vi "ReadSignals.Compile.vi"(8 "error in (no error)":errorcluster, 9 "Frame Settings Array":T4[](array[typedef]) {"Signals"."Byte Order" items=["Little Endian", "Big Endian"]; "Signals"."Data Type" items=["Signed", "Unsigned", "IEEE Float"]}, 10 "Refs":T3[](array[typedef]) {"Signal Refs" format="%.0x"}, 11 "Lookups in":variant) -> (0 "error out":errorcluster, 2 "Refs":T2 {"VS Refs" format="%.0x"}, 3 "Lookups":variant)   [LabVIEW 2019, in "Diagnostics Addon System Explorer.lvlib"]
uses:
  Diagnostics Addon System Explorer.lvlib
  Shared/Types/Frame.Compile.ctl
  Shared/Types/Type.ctl
  Shared/Types/Signal.ctl
  Types/Frame.Ref.ctl
  <vilib>/NI VeriStand/Custom Device API/Custom Device Item Ref.ctl
  Shared/Types/Frame.Lookup.Info.ctl
  Shared/SubVIs/Constants.vi
  Shared/Diagnostics Addon Shared.lvlib
  <vilib>/NI VeriStand/Custom Device API/Custom Device API.lvlib
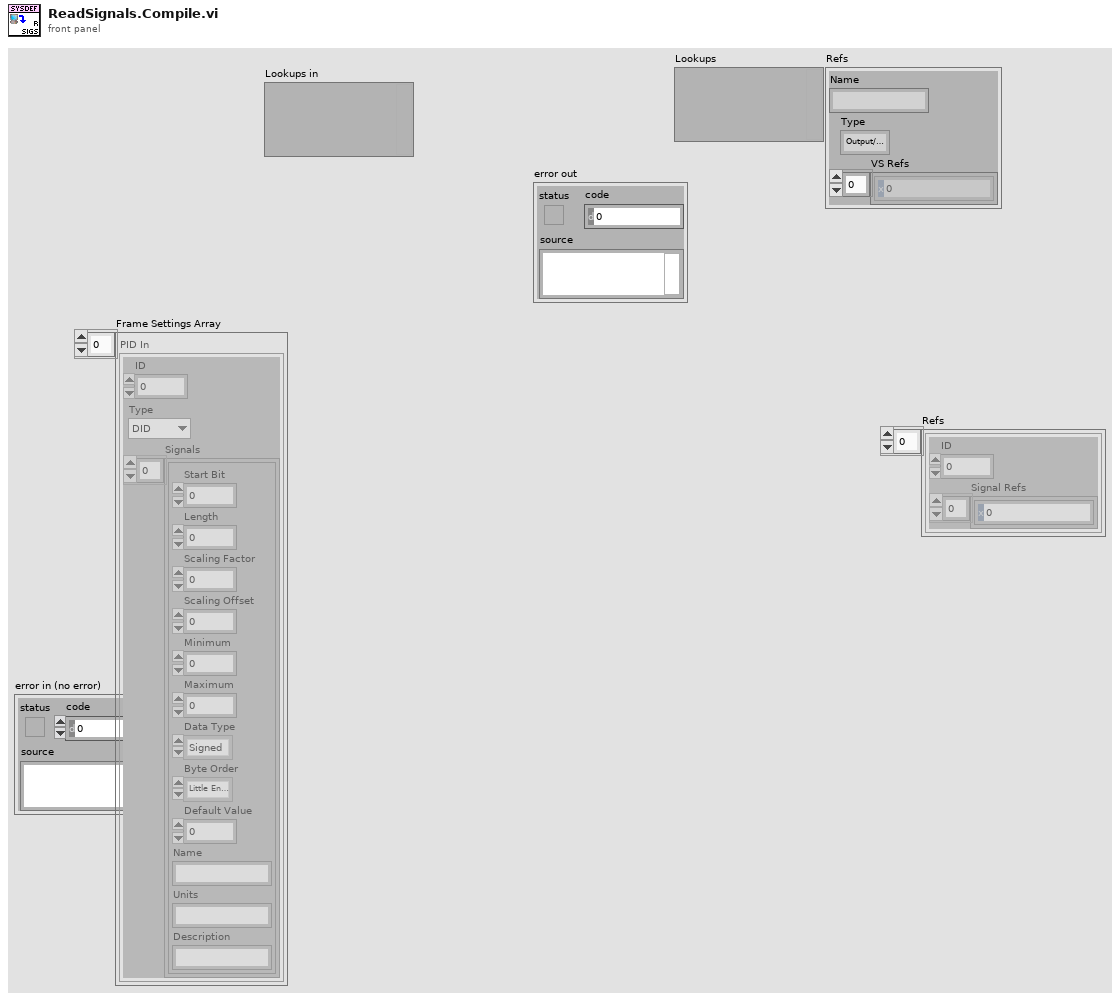
[diagram p1: front panel]
types:
  T1 = typedef "Custom Device API.lvlib/Custom Device Item Ref.ctl" = u64
  T2 = cluster{"Name":string, "Type":enum16{"Output/Write", "Input/Read", "Input/ReadWrite"}, "VS Refs":T1[]}
  T3 = typedef "Diagnostics Addon System Explorer.lvlib/Frame.Ref.ctl" = cluster{"ID":u32, "Signal Refs":T1[]}
  T4 = typedef "Diagnostics Addon Shared.lvlib/Frame.Compile.ctl" = cluster{"ID":u32, "Type":T5, "Signals":T6[]}
  T5 = typedef "Diagnostics Addon Shared.lvlib/Type.ctl" = enum16{"DID", "CDID", "PID", "CPID", "Read Memory", "Write Memory", "DTC Control", "IO Cmd", "IO Resp", "Routine Start Cmd", "Routine Start Resp", "Routine Request Cmd", "Routine Request Resp", "Routine Stop Cmd", "Routine Stop Resp", "UserDefined Cmd", "UserDefined Rsp"}
  T6 = typedef "Diagnostics Addon Shared.lvlib/Signal.ctl" = cluster{"Start Bit":u32, "Length":u32, "Scaling Factor":dbl, "Scaling Offset":dbl, "Minimum":dbl, "Maximum":dbl, "Data Type":u32, "Byte Order":u32, "Default Value":dbl, "Name":string, "Units":string, "Description":string}
  T7 = enum16{"Output/Write", "Input/Read", "Input/ReadWrite"}
  T8 = typedef "Diagnostics Addon Shared.lvlib/Frame.Lookup.Info.ctl" = cluster{"Offset":i32, "Length":i32, "ByteLength":u16}
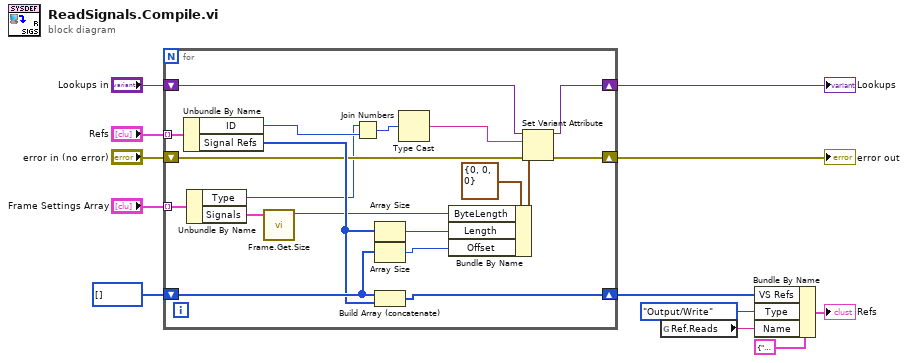
[diagram p0: block diagram]
diagram:
  n1 = for {
    tunnel: "Refs" -> [w21] mode=indexing
    shift-right: [w30] -> w3
    shift-left: T1[] [] ("Signal Refs") -> [w31]
    shift-right: [w22] -> w10
    shift-left: "Lookups in" -> [w26]
    shift-right: [w24] -> w1
    shift-left: "error in (no error)" -> [w19]
    tunnel: "Frame Settings Array" -> [w18] mode=indexing
    n2 = Unbundle By Name(w21) -> ("ID"=w15:u32, "Signal Refs"=w20:T1[])
    n3 = Unbundle By Name(w18) -> ("Type"=w13:T5, "Signals"=w17:T6[])
    n4 = call "Frame.Get.Size.vi"("Parameters"=w17) -> ("Bytes"=w16:u32)  [unwired: 10 in]
    n5 = Join Numbers(hi=w13, lo=w15) -> ((hi.lo)=w14:u64)
    n6 = Array Size(array=w20) -> (size(s)=w29:i32)
    n7 = Array Size(array=w31) -> (size(s)=w25:i32)
    n8 = Build Array (concatenate)(w31, w20) -> (w30:T1[])
    n9 = Type Cast(x=w14) -> (*(type *) &x=w23:string)  [unwired: 1 in]
    n10 = Bundle By Name(cluster=T8 {"Offset"=0, "Length"=0, "ByteLength"=0}, "ByteLength"=w16, "Length"=w29, "Offset"=w25) -> (w27:T8)
    n11 = Set Variant Attribute(Variant=w26, name=w23, value=w27, error in=w19) -> (Variant out=w22:variant, error out=w24:errorcluster)  [unwired: 1 out]
  }
  "error out" <- w1
  "Lookups" <- w10
  n12 = global read "Constants.vi" "Ref.Reads"() -> (w5:string)
  n13 = Bundle By Name(cluster=T2 {"Name"="", "Type"=enum."Output/Write", "VS Refs"=[]} ("Group"), "VS Refs"=w3, "Type"=T7."Output/Write", "Name"=w5) -> (→"Refs":T2)
